vi "timestamp_to_iso8601_string.vi"(9 "UTC? (T)":bool=TRUE, 10 "Time Stamp (now)":timestamp format="%<%x %.3X>T") -> (2 "ISO8601 UTC DateTime":string)   [LabVIEW 2020, in "Nominal Client.lvclass"]
doc: "Converts a LabVIEW timestamp into a standardized ISO8601 date-time string."
uses:
  Nominal Client.lvclass
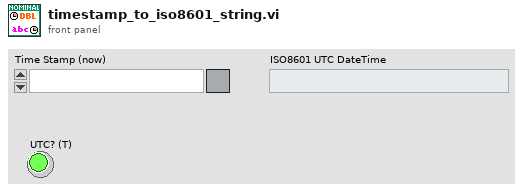
[diagram p1: front panel]
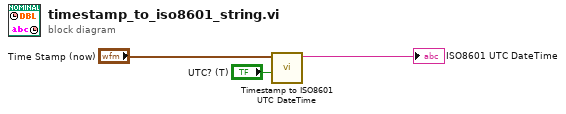
[diagram p0: block diagram]
diagram:
  n1 = call <vilib>:"Timestamp to ISO8601 UTC DateTime.vi"("UTC? (F)"="UTC? (T)", "Timestamp (now)"="Time Stamp (now)") -> ("ISO8601 UTC DateTime"=→"ISO8601 UTC DateTime":string)  [unwired: 9 in]
